vi "Configure Digital Pins.vi"(7 "Digital Pin Polarity (0: Positive)":u16(ring) items=["Positive", "Negative"], 8 "error in (no error)":errorcluster, 9 "Digital Pin Type (0: Input/Output)":u16(ring) items=["Input/Output", "Input Only", "Fault", "Inhibit", "Sync On", "Sync Off", "Trigger Input", "Trigger Output"], 10 "Pin Number (1)":u16=1, 11 "VISA resource name":refnum<visa-resource-name>) -> (0 "error out":errorcluster, 3 "VISA resource name out":refnum<visa-resource-name>)   [LabVIEW 2021, in "Agilent N6900 N7900 Series.lvlib"]
doc: "Configures any of the digital pins to a certain function amd polarity."
uses:
  <instrlib>/Agilent N6900 N7900 Series/Agilent N6900 N7900 Series.lvlib
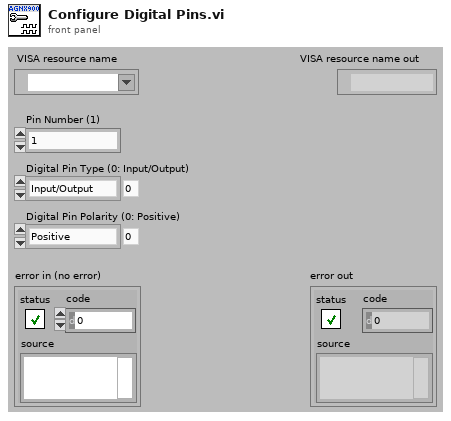
[diagram p1: front panel]
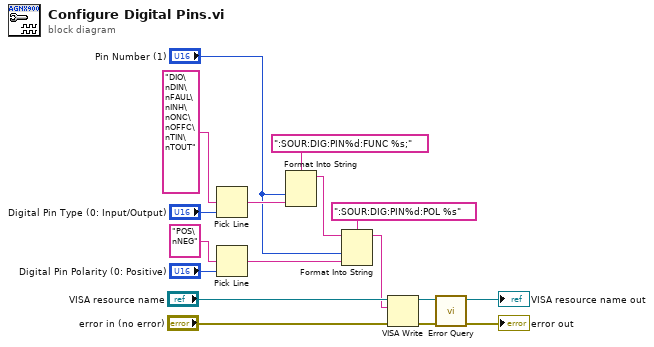
[diagram p0: block diagram]
diagram:
  n1 = Pick Line(multi-line string="DIO\nDIN\nFAUL\nINH\nONC\nOFFC\nTIN\nTOUT", line index="Digital Pin Type (0: Input/Output)") -> (output string=w8:string)  [unwired: 1 in]
  n2 = Pick Line(multi-line string="POS\nNEG", line index="Digital Pin Polarity (0: Positive)") -> (output string=w4:string)  [unwired: 1 in]
  n3 = Format Into String(format string=":SOUR:DIG:PIN%d:FUNC %s;", "Pin Number (1)", w8) -> (resulting string=w1:string)  [unwired: 2 in, 1 out]
  n4 = Format Into String(format string=":SOUR:DIG:PIN%d:POL %s", initial string=w1, "Pin Number (1)", w4) -> (resulting string=w2:string)  [unwired: 1 in, 1 out]
  n5 = VISA Write(VISA resource name="VISA resource name", write buffer=w2, error in (no error)="error in (no error)") -> (VISA resource name out=w15:refnum<visa-resource-name>, error out=w16:errorcluster)  [unwired: 1 out]
  n6 = call <instrlib>:"Error Query.vi"("error in (no error)"=w16, "VISA resource name"=w15) -> ("error out"=→"error out":errorcluster, "VISA resource name out"=→"VISA resource name out":refnum<visa-resource-name>)  [unwired: 6 in, 2 out]
